vi "05TRM800_PartNum.vi"(8 "error in (no error)":errorcluster, 10 "Input":string, 11 "Enum":enum16{"Initialize", "Get", "Input"}(ring)) -> (0 "error out":errorcluster, 3 "Part Num":string)   [LabVIEW 2020]
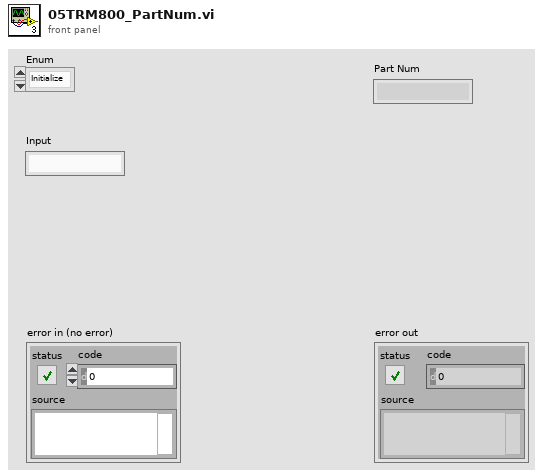
[diagram p1: front panel]
types:
  T1 = enum16{"Initialize", "Next", "Send RSET", "Set MPH", "Set INC", "Part to 0"}
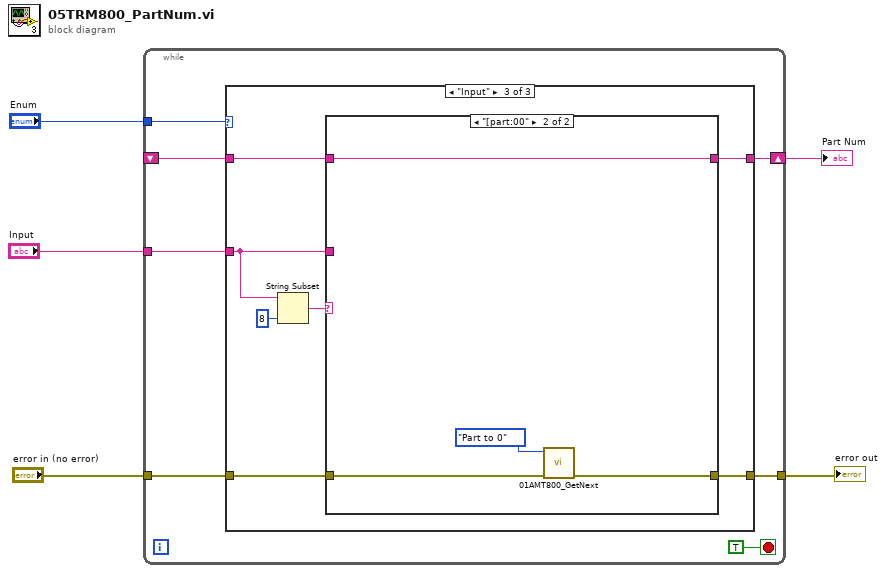
[diagram p0: block diagram]
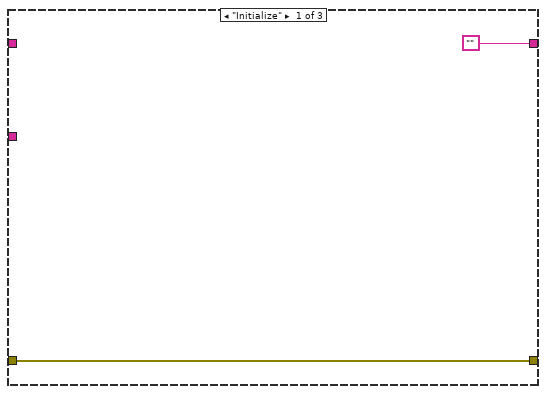
[diagram p2: hidden frame]
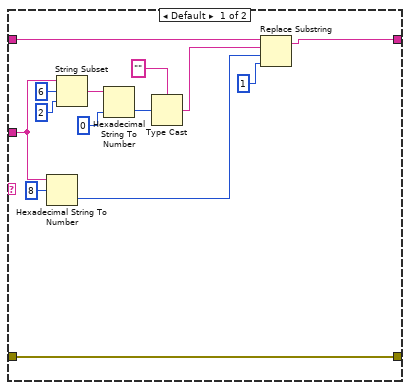
[diagram p4: hidden frame]
diagram:
  n1 = while {
    tunnel: "error in (no error)" -> [w10]
    tunnel: "Enum" -> [w11]
    tunnel: [w9] -> w3
    tunnel: "Input" -> [w8]
    shift-right: [w7] -> w1
    shift-left: _ -> [w6]
    stop <- TRUE stop-if-true
    n2 = case shown="\"Input\"" w11 {
      tunnel: w10 -> [w13 w16 w21]
      tunnel: [w13 w16 w20] -> w9
      tunnel: w8 -> [_ _ w17]
      tunnel: ["" w15 w18] -> w7
      tunnel: w6 -> [_ w15 w19]
      frame "Initialize" {
      }
      frame "Get" {
      }
      frame "Input" {
        n3 = String Subset(string=w17, length (rest)=8 ("length (rest)")) -> (substring=w22:string)  [unwired: 1 in]
        n4 = case shown="\"[part:00\"" w22 {
          tunnel: w21 -> [w37 w41]
          tunnel: [w37 w40] -> w20
          tunnel: w19 -> [w34 w38]
          tunnel: [w33 w38] -> w18
          tunnel: w17 -> [w31 _]
          frame Default {
            n5 = Hexadecimal String To Number(string=w31, offset=8) -> (number=w35:u32)  [unwired: 1 in, 1 out]
            n6 = String Subset(string=w31, offset (0)=6, length (rest)=2 ("length (rest)")) -> (substring=w28:string)
            n7 = Hexadecimal String To Number(string=w28, default (0uL)=u8 0 ("default (0 U32)")) -> (number=w26:u8)  [unwired: 1 in, 1 out]
            n8 = Type Cast(type="", x=w26) -> (*(type *) &x=w24:string)
            n9 = Replace Substring(2:1 ("length (len. of substring)"), 3:w35, 4:w24, 5:w34) -> (1:w33:string)  [unwired: 1 out]
          }
          frame "[part:00" {
            n10 = call "01AMT800_GetNext.vi"("error in (no error)"=w41, "Enum"=T1."Part to 0") -> ("error out"=w40:errorcluster)  [unwired: 8 in, 1 out]
          }
        }
      }
    }
  }
  "error out" <- w3
  "Part Num" <- w1
